vi "Split.vi"(8 "error in":errorcluster caption="错误输入（无错误）", 10 "Data":variant, 11 "PanelRootNode 输入":refnum<class "PanelRootNode.lvclass"> caption="DNL_LabVIEW Object in") -> (0 "error out":errorcluster caption="错误输出", 3 "PanelRootNode 输出":refnum<class "PanelRootNode.lvclass"> caption="DNL_LabVIEW Object out")   [LabVIEW 2013, in "PanelRootNode.lvclass"]
doc: "本VI作用为分割目标窗格。\n变体Data为含有两个元素的簇，簇中第二个元素为分割模式（横向、纵向等），\n第一个元素可有三种形式：\n1.Node*\n2.Panel Number\n3.Node Path"
uses:
  PanelRootNode.lvclass
  PanelObject/PanelObject.lvclass
  PanelDataNode/Split Mode.ctl
  PanelDataNode/PanelDataNode.lvclass
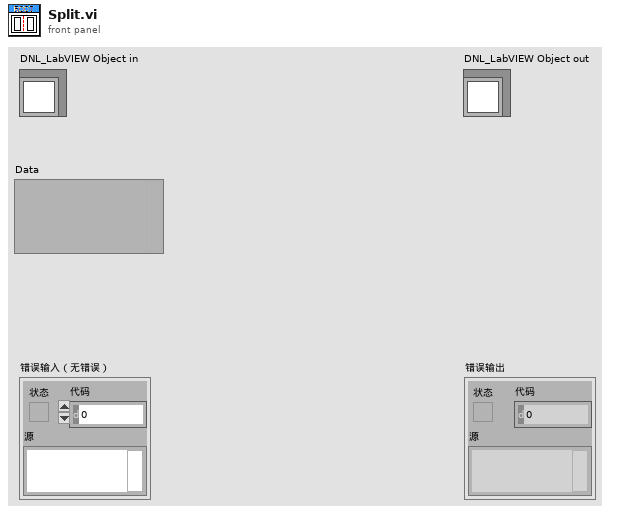
[diagram p1: front panel]
types:
  T1 = typedef "PanelDataNode.lvclass/Split Mode.ctl" = enum16{"Horizontal(up)", "Vertical(left)", "Horizontal(down)", "Vertical(right)"}
  T2 = cluster{"Node*":refnum<data-value>, "Split Mode":T1}
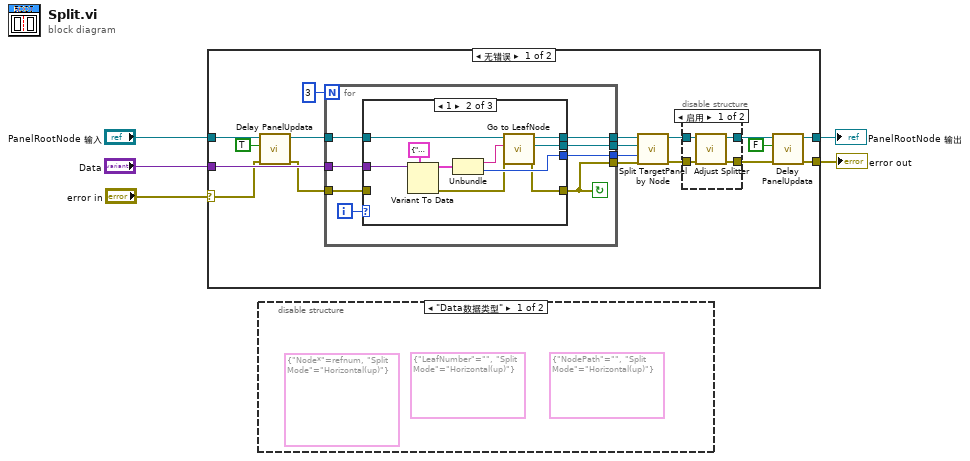
[diagram p0: block diagram]
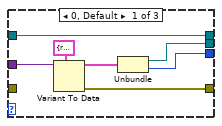
[diagram p4: hidden frame]
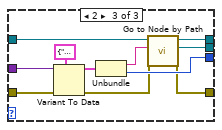
[diagram p5: hidden frame]
diagram:
  n1 = case shown="无错误" "error in" {
    selector: "error in" -> [w15 w67]
    tunnel: [w11 w67] -> w4
    tunnel: [w12 w66] -> w2
    tunnel: "PanelRootNode 输入" -> [w17 w66]
    tunnel: "Data" -> [w18 _]
    frame No Error {
      n2 = call "Delay PanelUpdata.vi"("error in (no error)"=w15, "延迟前面板更新"=TRUE, "PanelRootNode 输入"=w17) -> ("error out"=w14:errorcluster, "PanelRootNode 输出"=w16:refnum<class "PanelRootNode.lvclass">)  [unwired: 7 in]
      n3 = for {
        N: 3 -> [_]
        tunnel: [w36] -> w22
        tunnel: [w35] -> w21
        tunnel: w16 -> [w34]
        tunnel: [w33] -> w20
        tunnel: [w32] -> w19
        tunnel: w18 -> [w31]
        tunnel: w14 -> [w30]
        i -> [w37]
        stop <- w32 continue-if-true
        n4 = case shown="1" w37 {
          tunnel: [w44 w54 w65] -> w33
          tunnel: [w43 w49 w60] -> w35
          tunnel: [w39 w52 w62] -> w36
          tunnel: [w40 w48 w59] -> w32
          tunnel: w34 -> [w39 w46 w58]
          tunnel: w31 -> [w38 w45 w56]
          tunnel: w30 -> [_ _ w55]
          frame 0, Default {
            n5 = Variant To Data(type=T2 {"Node*"=refnum, "Split Mode"=enum."Horizontal(up)"}, Variant=w38) -> (data=w42:T2, error out=w40:errorcluster)  [unwired: 1 in]
            n6 = Unbundle(w42) -> ("Node*"=w43:refnum<data-value>, "Split Mode"=w44:T1)
          }
          frame 1 {
            n7 = Variant To Data(type=cluster{string, "Split Mode":T1} {"", "Split Mode"=enum."Horizontal(up)"}, Variant=w45) -> (data=w53:cluster{string, "Split Mode":T1}, error out=w47:errorcluster)  [unwired: 1 in]
            n8 = Unbundle(w53) -> (w50:string, "Split Mode"=w54:T1)
            n9 = call-dynamic "Go to LeafNode.vi"("error in"=w47, "LeafNumber"=w50, "PanelRootNode 输入"=w46) -> ("error out"=w48:errorcluster, "Node*"=w49:refnum<data-value>, "PanelRootNode 输出"=w52:refnum<class "PanelRootNode.lvclass">)  [unwired: 5 in, 1 out]
          }
          frame 2 {
            n10 = Variant To Data(error in=w55, type=cluster{string, "Split Mode":T1} {"", "Split Mode"=enum."Horizontal(up)"}, Variant=w56) -> (data=w64:cluster{string, "Split Mode":T1}, error out=w57:errorcluster)
            n11 = Unbundle(w64) -> (w61:string, "Split Mode"=w65:T1)
            n12 = call-dynamic "Go to Node by Path.vi"("error in"=w57, "NodePath"=w61, "PanelLinkNode 输入"=w58) -> ("error out"=w59:errorcluster, "Node*"=w60:refnum<data-value>, "PanelLinkNode 输出"=w62:refnum<class "PanelRootNode.lvclass">)  [unwired: 5 in, 1 out]
          }
        }
      }
      n13 = call-dynamic "Split TargetPanel by Node.vi"("error in"=w19, "Split Mode"=w20, "Node*"=w21, "PanelRootNode 输入"=w22) -> ("error out"=w7:errorcluster, "PanelRootNode 输出"=w9:refnum<class "PanelRootNode.lvclass">)  [unwired: 5 in, 1 out]
      n14 = disable-structure shown="启用" {
        disable-tunnel: w9 -> [w27 w29]
        disable-tunnel: [w26 w29] -> w8
        disable-tunnel: w7 -> [w25 w28]
        disable-tunnel: [w24 w28] -> w6
        frame Enabled {
          n15 = call "Adjust Splitter.vi"("error in (no error)"=w25, "PanelRootNode 输入"=w27) -> ("error out"=w24:errorcluster, "PanelRootNode 输出"=w26:refnum<class "PanelRootNode.lvclass">)  [unwired: 8 in]
        }
        frame Disabled {
        }
      }
      n16 = call "Delay PanelUpdata.vi"("error in (no error)"=w6, "延迟前面板更新"=FALSE, "PanelRootNode 输入"=w8) -> ("error out"=w11:errorcluster, "PanelRootNode 输出"=w12:refnum<class "PanelRootNode.lvclass">)  [unwired: 7 in]
    }
    frame Error {
    }
  }
  "error out" <- w4
  "PanelRootNode 输出" <- w2
  n17 = disable-structure shown="\"Data数据类型\"" {
    frame condition #0 {
      (unwired) cluster{"NodePath":string, "Split Mode":T1} {"NodePath"="", "Split Mode"=enum."Horizontal(up)"}
      (unwired) cluster{"LeafNumber":string, "Split Mode":T1} {"LeafNumber"="", "Split Mode"=enum."Horizontal(up)"}
      (unwired) T2 {"Node*"=refnum, "Split Mode"=enum."Horizontal(up)"}
    }
    frame condition #1 (active) {
    }
  }
